vi "fpga_cont_det.vi"(0 "X":fxp<+/-,24,5>, 1 "X Center":fxp<+/-,24,5>, 2 "Min Angle 2":fxp<+,9,9>=1.0 format="%.52g", 3 "Y":fxp<+/-,24,5>, 4 "Y Center":fxp<+/-,24,5>, 5 "Touch 1":bool, 6 "Nose Poke":bool, 7 "Touch 2":bool, 8 "Threshold":fxp<+,22,9>, 9 "Flip 1":bool, 10 "Max Angle 2":fxp<+,9,9> format="%.52g", 11 "CCW(T)":bool, 12 "Max Angle":fxp<+,9,9> format="%.52g", 13 "Flip 2":bool, 14 "Min Angle":fxp<+,9,9>=1.0 format="%.52g", 15 "Flip XY":bool, 16 "CCW(T)  2":bool, 17 "Radius Voltage":fxp<+/-,24,5>, 18 "Laser ?":bool) -> (20 "Contingency":bool, 21 "Deviation":fxp<+,22,10>, 23 "X":fxp<+/-,22,10> format="%.16g", 24 "Y":fxp<+/-,22,10> format="%.16g", 25 "angle":fxp<+/-,9,9>, 27 "angle_out":bool)   [LabVIEW 2013]
doc: "Determine if all contingencies have been met:\n1. Joystick moved far enough\n2. Angle within target range\n3. Touch 1 touched\n4. Touch 2 touched\n5. Nose poke occurred"
uses:
  <vilib>/rvi/FXPMathLib/FxpDiv/subVIs/nifxpmath_Div_SimConfig.ctl
  <vilib>/rvi/FXPMathLib/FxpRectToPolar/subVIs/nifxpmath_RectToPolar_SimConfig.ctl
  <vilib>/rvi/FXPMathLib/FxpDiv/simVIs/DllFxpDivTemp_sub.vi
  <vilib>/rvi/FXPMathLib/FxpRectToPolar/simVIs/DllFxpRectToPolarTemp_sub.vi
  <vilib>/rvi/FXPMathLib/FxpSub/XNode/nifxpmath_Sub.xnode
  <vilib>/rvi/FXPMathLib/FxpDiv/XNode/nifxpmath_Div.xnode
  <vilib>/rvi/FXPMathLib/FxpMul/XNode/nifxpmath_Multiplier.xnode
  <vilib>/rvi/FXPMathLib/FxpRectToPolar/XNode/nifxpmath_RectToPolar.xnode
  <vilib>/rvi/FXPMathLib/sim/FxpSim.dll
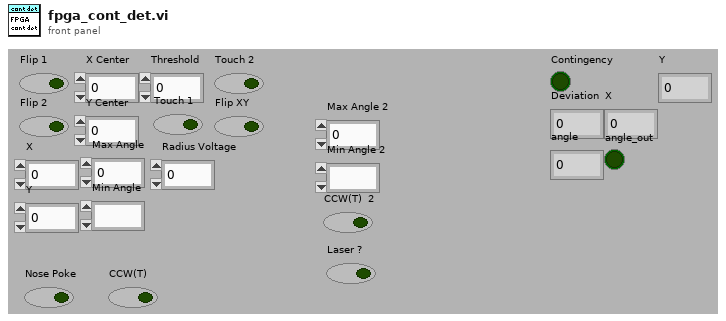
[diagram p1: front panel]
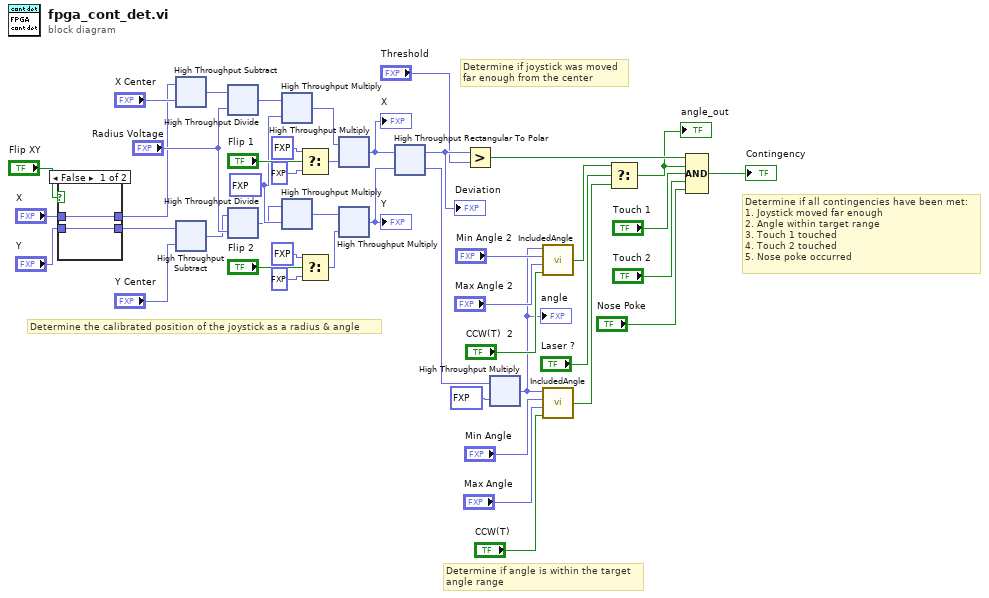
[diagram p0: block diagram]
diagram:
  w27 = fxp<+,5,7> 100.0
  # "Determine if all contingencies have been met:\n1. Joystick moved far enough\n2. Angle within target range\n3. Touch 1 touched\n4. Touch 2 touched\n5. Nose poke occurred"
  # "Determine if joystick was moved\nfar enough from the center"
  # "Determine if angle is within the target\nangle range"
  # "Determine the calibrated position of the joystick as a radius & angle"
  n1 = case shown="False" "Flip XY" {
    tunnel: [w46 w49] -> w19
    tunnel: "X" -> [w47 w49]
    tunnel: "Y" -> [w46 w48]
    tunnel: [w47 w48] -> w22
    frame False {
    }
    frame True {
    }
  }
  n2 = xnode "High Throughput Subtract"("x"=w22, "y"="X Center") -> ("x-y"=w21:fxp<+/-,24,5>)
  n3 = xnode "High Throughput Subtract"("x"=w19, "y"="Y Center") -> ("x-y"=w17:fxp<+/-,24,5>)
  n4 = xnode "High Throughput Divide"("x"=w21, "y"="Radius Voltage") -> ("x/y"=w26:fxp<+/-,24,5>)
  n5 = xnode "High Throughput Divide"("x"=w17, "y"="Radius Voltage") -> ("x/y"=w25:fxp<+/-,24,5>)
  n6 = xnode ("High Throughput Multiply")("x"=w26, "y"=w27) -> ("x*y"=w24:fxp<+/-,29,12>)
  n7 = xnode ("High Throughput Multiply")("x"=w25, "y"=w27) -> ("x*y"=w20:fxp<+/-,29,12>)
  n8 = Select(t=fxp<+/-,1,1> -1.0, s="Flip 1", f=fxp<+,1,1> 1.0) -> (s? t:f=w39:fxp<+/-,2,2>)
  n9 = Select(t=fxp<+/-,1,1> -1.0, s="Flip 2", f=fxp<+,1,1> 1.0) -> (s? t:f=w38:fxp<+/-,2,2>)
  n10 = xnode ("High Throughput Multiply")("x"=w24, "y"=w39) -> ("x*y"=w37:fxp<+/-,22,10>)
  "X" <- w37
  n11 = xnode ("High Throughput Multiply")("x"=w20, "y"=w38) -> ("x*y"=w36:fxp<+/-,22,10>)
  "Y" <- w36
  n12 = xnode "High Throughput Rectangular To Polar"("x"=w37, "y"=w36) -> ("magnitude"=w15:fxp<+,22,10>, "phase (pi)"=w35:fxp<+/-,13,2>)
  "Deviation" <- w15
  n13 = Greater?(x=w15, y="Threshold") -> (0:w13:bool)
  n14 = xnode ("High Throughput Multiply")("x"=w35, "y"=fxp<+,16,8> 180.0) -> ("x*y"=w5:fxp<+/-,9,9>)
  "angle" <- w5
  n15 = call "IncludedAngle.vi"("CCW(T)"="CCW(T)  2", "upper limit"="Max Angle 2", "lower limit"="Min Angle 2", "angle"=w5) -> ("s? t:f"=w3:bool)
  n16 = call "IncludedAngle.vi"("CCW(T)"="CCW(T)", "upper limit"="Max Angle", "lower limit"="Min Angle", "angle"=w5) -> ("s? t:f"=w4:bool)
  n17 = Select(t=w3, s="Laser ?", f=w4) -> (s? t:f=w2:bool)
  "angle_out" <- w2
  n18 = Compound Arithmetic op=AND(w13, w2, "Touch 1", "Touch 2", "Nose Poke") -> (→"Contingency":bool)
